vi "Acquisition Settings Dialog.vi"(8 "error in (no error)":errorcluster, 11 "Tasks in":T1[](array[typedef])) -> (0 "error out":errorcluster, 2 "cancelled":bool, 3 "Tasks out":T1[](array[typedef]))   [LabVIEW 2018, in "DAQ.lvlib"]
uses:
  Task Cluster (with Add Remove Buttons).ctl
  Task Cluster.ctl
  <vilib>/DAQmx/read.llb/DAQmx Read (Analog 1D Wfm NChan NSamp).vi
  <vilib>/DAQmx/miscellaneous.llb/DAQmx Fill In Error Info.vi
  DAQ/DAQ.lvlib
  <resource>/objmgr/daqmx.rc
panel:
  out "Channels":refnum<k21>[](array[refnum])
  out "error out 2":errorcluster
  in  "Cancel Button":bool
  in  "OK Button":bool
  in  "Task List":T2[](array[typedef]) caption="Channel List"
  # "DAQmx Tasks"
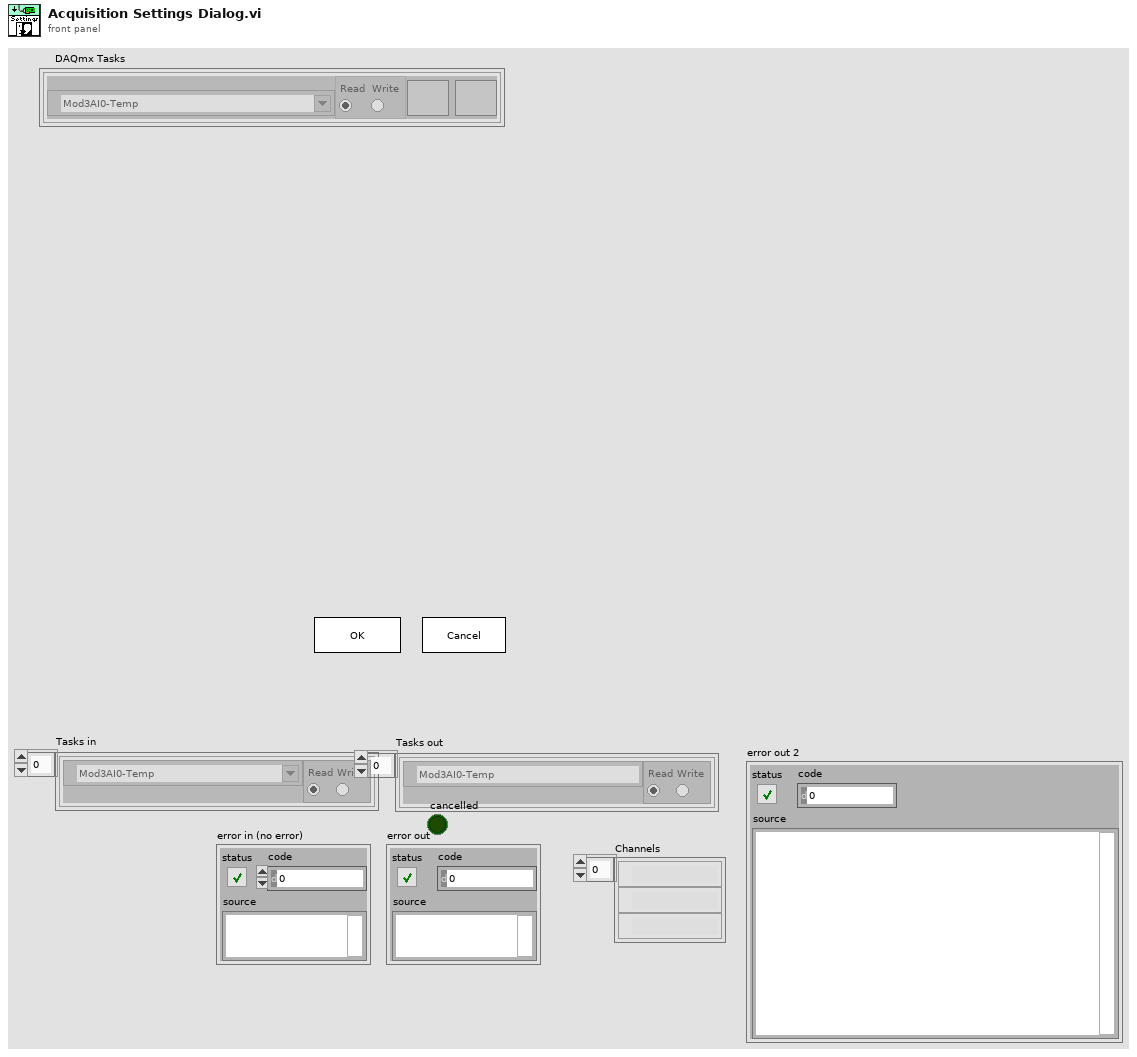
[diagram p1: front panel]
types:
  T1 = typedef "Task Cluster.ctl" = cluster{"DAQmx Task":refnum<k21>, "Read-Write Radio":enum32{"Read", "Write"}}
  T2 = typedef "DAQ.lvlib/Task Cluster (with Add Remove Buttons).ctl" = cluster{"Add Button":bool, "Remove Button":bool, "DAQmx Task":refnum<k21>, "Radio Buttons":enum32{"Read", "Write"}}
  T3 = enum8{"Enabled", "Disabled", "Disabled and Grayed Out"}
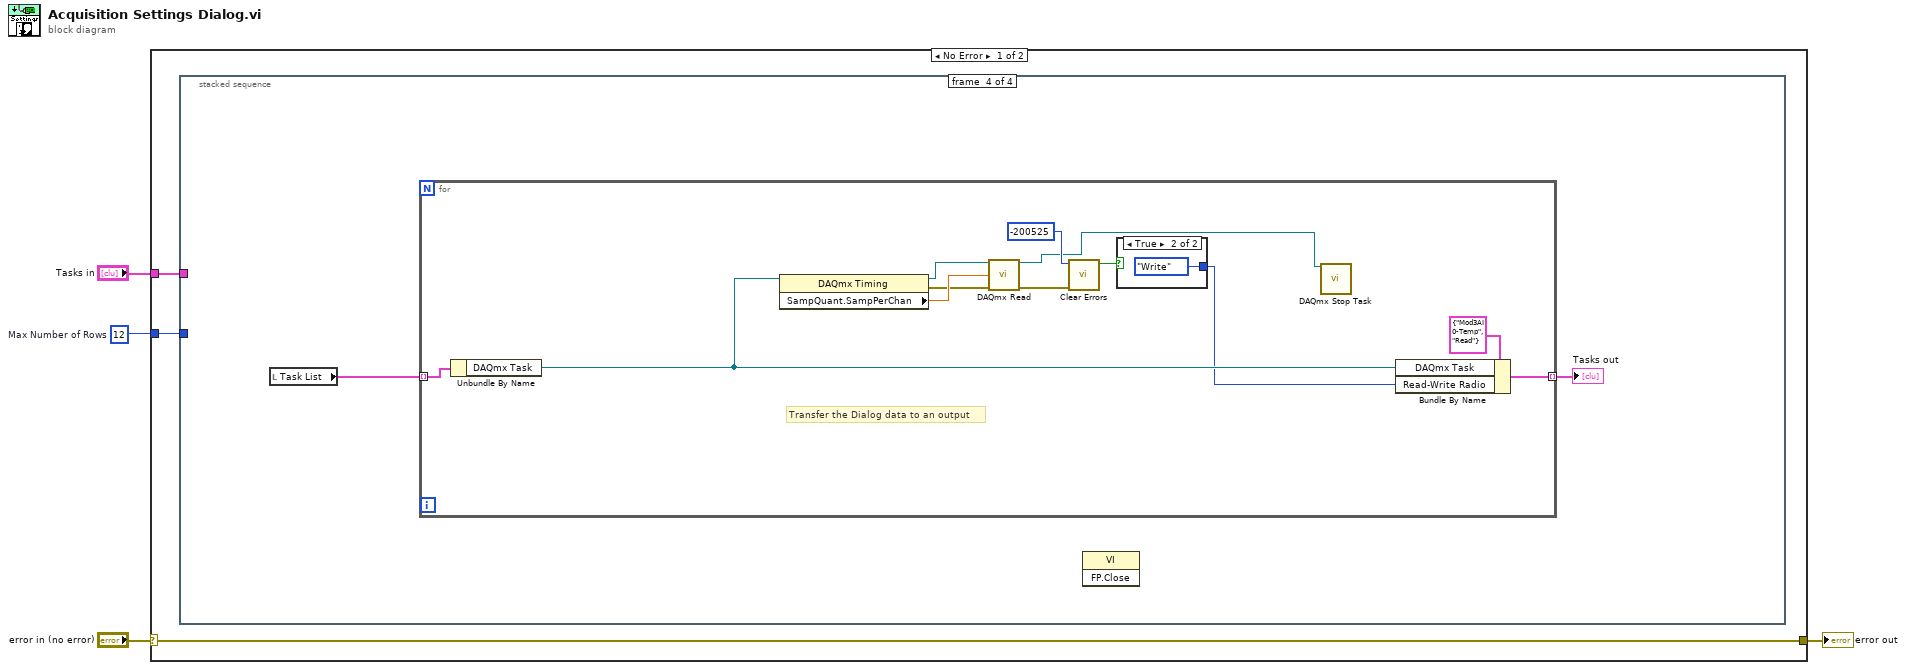
[diagram p0: block diagram]
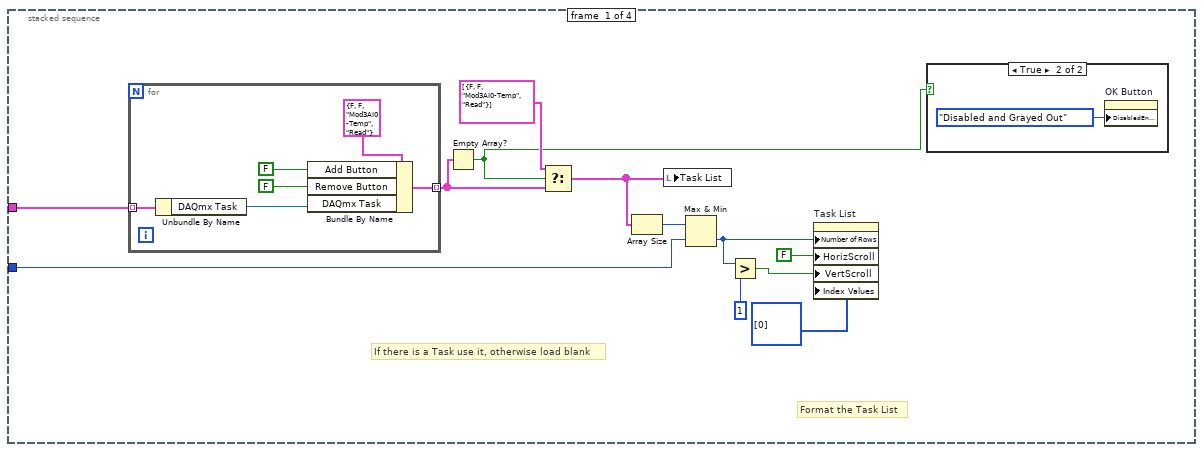
[diagram p2: hidden frame]
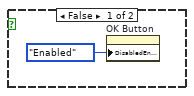
[diagram p3: hidden frame]
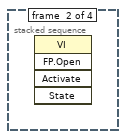
[diagram p4: hidden frame]
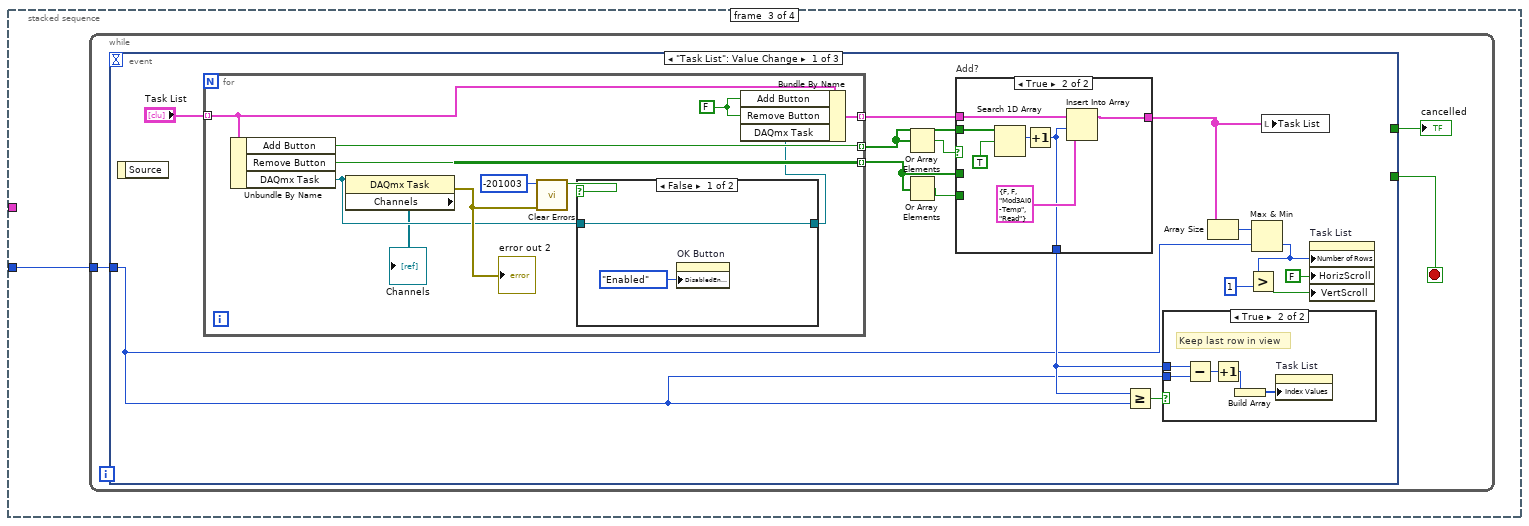
[diagram p5: hidden frame]
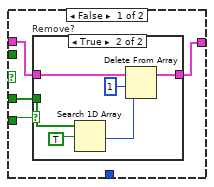
[diagram p7: hidden frame]
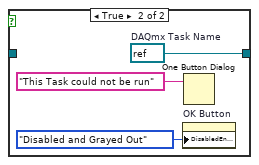
[diagram p9: hidden frame]
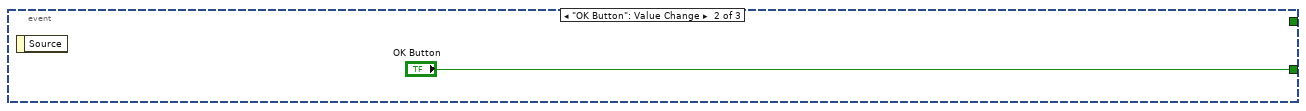
[diagram p10: hidden frame]
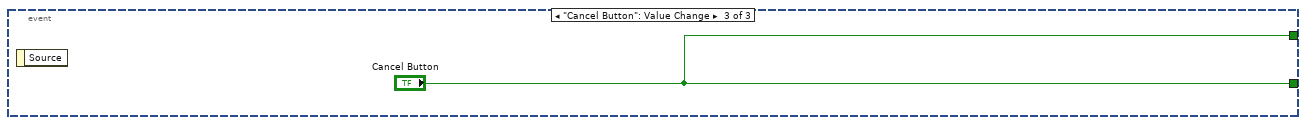
[diagram p11: hidden frame]
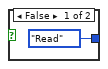
[diagram p12: hidden frame]
diagram:
  w1 = u32 12  # Max Number of Rows
  n1 = case shown="No Error" "error in (no error)" {
    selector: "error in (no error)" -> [w7 w104]
    tunnel: [w7 w104] -> w3
    tunnel: "Tasks in" -> [w6 _]
    tunnel: w1 -> [w5 _]
    frame No Error {
      n2 = stacked-sequence {
        tunnel: w6 -> [w19 _ _ _]
        tunnel: w5 -> [w14 _ w28 _]
        frame #0 {
          # "Format the Task List"
          # "If there is a Task use it, otherwise load blank"
          n3 = for {
            tunnel: w19 -> [w27] mode=indexing
            tunnel: [w22] -> w17 mode=indexing
            n4 = Unbundle By Name(w27) -> ("DAQmx Task"=w24:refnum<k21>)
            n5 = Bundle By Name(cluster=T2 {"Add Button"=FALSE, "Remove Button"=FALSE, "DAQmx Task"="Mod3AI0-Temp", "Radio Buttons"=enum."Read"} ("DAQmx Channel Cluster"), "Add Button"=FALSE, "Remove Button"=FALSE, "DAQmx Task"=w24) -> (w22:T2)
          }
          n6 = Empty Array?(array=w17) -> (empty?=w8:bool)
          n7 = Select(t=T2[] [{"Add Button"=FALSE, "Remove Button"=FALSE, "DAQmx Task"="Mod3AI0-Temp", "Radio Buttons"=enum."Read"}] ("Channel List"), s=w8, f=w17) -> (s? t:f=w16:T2[])
          n8 = Array Size(array=w16) -> (size(s)=w15:i32)
          n9 = local write "Task List"(w16) -> ()
          n10 = Max & Min(x=w15, y=w14) -> (min(x,y)=w12:u32)  [unwired: 1 out]
          n11 = Greater?(x=w12, y=u32 1) -> (0:w10:bool)
          n12 = property on="Task List" class="Arr"("Number of Rows"=w12, "HorizScroll"=FALSE ("Horizontal Scrollbar Visible"), "VertScroll"=w10, "Index Values"=u32[] [0]) -> ()  [unwired: 2 in, 2 out]
          n13 = case shown="True" w8 {
            frame False {
              n14 = property on="OK Button" class="Bool"("DisabledEnum"=T3."Enabled" ("Disabled")) -> ()  [unwired: 2 in, 2 out]
            }
            frame True {
              n15 = property on="OK Button" class="Bool"("DisabledEnum"=T3."Disabled and Grayed Out" ("Disabled")) -> ()  [unwired: 2 in, 2 out]
            }
          }
        }
        frame #1 {
          n16 = invoke class="VI" method="FP.Open"() -> ()  [unwired: 5 in, 5 out]
        }
        frame #2 {
          n17 = while {
            tunnel: w28 -> [w31]
            stop <- w30 stop-if-true
            n18 = event shown="[0] \"Task List\": Value Change" {
              selector: _ -> [_ _ _]
              dyn-events: _ -> [_ _ _]
              timeout: _ -> [_ _ _]
              tunnel: [_ "OK Button" "Cancel Button"] -> w30
              tunnel: w31 -> [w32 _ _]
              tunnel: [_ _ "Cancel Button"] -> w29
              event "Task List": Value Change {
                n19 = event-data() -> ()  [unwired: 1 in, 1 out]
                n20 = for {
                  tunnel: "Task List" -> [w79] mode=indexing
                  tunnel: [w76] -> w44 mode=indexing
                  tunnel: [w80] -> w42 mode=indexing
                  tunnel: [w77] -> w43 mode=indexing
                  w78 = FALSE ("Add Button")
                  n21 = Unbundle By Name(w79) -> ("Add Button"=w76:bool, "Remove Button"=w80:bool, "DAQmx Task"=w72:refnum<k21>)
                  n22 = property class="DAQmx Task"(reference=w72) -> (error out=w75:errorcluster, "Channels"=→"Channels":refnum<k21>[])  [unwired: 1 in, 1 out]
                  "error out 2" <- w75
                  n23 = call <vilib>:"Clear Errors.vi"("error in (no error)"=w75, "specific error code to clear (0: all)"=-201003) -> ("specific error cleared?"=w73:bool)  [unwired: 4 in, 1 out]
                  n24 = case shown="False" w73 {
                    tunnel: w72 -> [w82 _]
                    tunnel: [w82 w85] -> w71
                    frame False {
                      n25 = property on="OK Button" class="Bool"("DisabledEnum"=T3."Enabled" ("Disabled")) -> ()  [unwired: 2 in, 2 out]
                    }
                    frame True {
                      w85 = refnum<k21> refnum  # DAQmx Task Name
                      n26 = property on="OK Button" class="Bool"("DisabledEnum"=T3."Disabled and Grayed Out" ("Disabled")) -> ()  [unwired: 2 in, 2 out]
                      n27 = One Button Dialog(message="This Task could not be run") -> ()  [unwired: 1 in, 1 out]
                    }
                  }
                  n28 = Bundle By Name(cluster=w79, "Add Button"=w78, "Remove Button"=w78, "DAQmx Task"=w71) -> (w77:T2)
                }
                n29 = Or Array Elements(Boolean array=w44) -> (logical OR=w45:bool)
                n30 = Or Array Elements(Boolean array=w42) -> (logical OR=w41:bool)
                n31 = case "Add?" shown="True" w45 {
                  tunnel: w44 -> [_ w69]
                  tunnel: w43 -> [w53 w67]
                  tunnel: [w52 w64] -> w40
                  tunnel: w42 -> [w55 _]
                  tunnel: w41 -> [w54 _]
                  tunnel: [_ w63] -> w33
                  frame False {
                    n32 = case "Remove?" shown="True" w54 {
                      tunnel: w55 -> [_ w61]
                      tunnel: w53 -> [w56 w60]
                      tunnel: [w56 w57] -> w52
                      frame False {
                      }
                      frame True {
                        n33 = Search 1D Array(1D array=w61, element=TRUE) -> (index of element=w58:i32)  [unwired: 1 in]
                        n34 = Delete From Array(array=w60, length=1, index=w58) -> (array with subset deleted=w57:T2[])  [unwired: 1 out]
                      }
                    }
                  }
                  frame True {
                    n35 = Search 1D Array(1D array=w69, element=TRUE) -> (index of element=w66:i32)  [unwired: 1 in]
                    n36 = Increment(x=w66) -> (x+1=w63:i32)
                    n37 = Insert Into Array(array=w67, index=w63, new element=T2 {"Add Button"=FALSE, "Remove Button"=FALSE, "DAQmx Task"="Mod3AI0-Temp", "Radio Buttons"=enum."Read"} ("new element/subarray")) -> (w64:T2[])
                  }
                }
                n38 = Greater Or Equal?(x=w33, y=w32) -> (x >= y?=w34:bool)
                n39 = case shown="True" w34 {
                  tunnel: w33 -> [_ w51]
                  tunnel: w32 -> [_ w50]
                  frame False {
                  }
                  frame True {
                    # "Keep last row in view"
                    n40 = Subtract(x=w51, y=w50) -> (x-y=w49:u32)
                    n41 = Increment(x=w49) -> (x+1=w47:u32)
                    n42 = Build Array(w47) -> (w48:u32[])
                    n43 = property on="Task List" class="Arr"("Index Values"=w48) -> ()  [unwired: 2 in, 2 out]
                  }
                }
                n44 = Array Size(array=w40) -> (size(s)=w39:i32)
                n45 = Max & Min(x=w39, y=w32) -> (min(x,y)=w36:u32)  [unwired: 1 out]
                n46 = Greater?(x=w36, y=u32 1) -> (0:w35:bool)
                n47 = local write "Task List"(w40) -> ()
                n48 = property on="Task List" class="Arr"("Number of Rows"=w36, "HorizScroll"=FALSE ("Horizontal Scrollbar Visible"), "VertScroll"=w35) -> ()  [unwired: 2 in, 2 out]
              }
              event "OK Button": Value Change {
                n49 = event-data() -> ()  [unwired: 1 in, 1 out]
              }
              event "Cancel Button": Value Change {
                n50 = event-data() -> ()  [unwired: 1 in, 1 out]
              }
            }
            "cancelled" <- w29
          }
        }
        frame #3 {
          n51 = local read "Task List"() -> (w89:T2[])
          n52 = for {
            tunnel: w89 -> [w99] mode=indexing
            tunnel: [w100] -> w88 mode=indexing
            # "Transfer the Dialog data to an output"
            n53 = Unbundle By Name(w99) -> ("DAQmx Task"=w101:refnum<k21>)
            n54 = property class="DAQmx Timing"(reference=w101) -> (reference out=w93:refnum<k21>, error out=w94:errorcluster, "SampQuant.SampPerChan"=w95:dbl)  [unwired: 1 in]
            n55 = call-poly <vilib>:"DAQmx Read.vi"("task/channels in"=w93, "number of samples per channel"=w95, "error in"=w94) -> ("task out"=w90:refnum<k21>, "error out"=w97:errorcluster)  [unwired: 10 in, 1 out]
            n56 = call <vilib>:"Clear Errors.vi"("error in (no error)"=w97, "specific error code to clear (0: all)"=-200525) -> ("specific error cleared?"=w96:bool)  [unwired: 4 in, 1 out]
            n57 = case shown="True" w96 {
              tunnel: [enum32{"Read", "Write"}."Read" ("Read-Write Radio") enum32{"Read", "Write"}."Write" ("Read-Write Radio")] -> w91
              frame False {
              }
              frame True {
              }
            }
            n58 = call <vilib>:"DAQmx Stop Task.vi"("task/channels in"=w90) -> ()  [unwired: 13 in, 2 out]
            n59 = Bundle By Name(cluster=T1 {"DAQmx Task"="Mod3AI0-Temp", "Read-Write Radio"=enum."Read"} ("DAQmx Channel Cluster"), "DAQmx Task"=w101, "Read-Write Radio"=w91) -> (w100:T1)
          }
          "Tasks out" <- w88
          n60 = invoke class="VI" method="FP.Close"() -> ()  [unwired: 3 in, 3 out]
        }
      }
    }
    frame Error {
    }
  }
  "error out" <- w3
